vi "RFmxSpecAn Get Results Deployed(Harms).vi"(0 "SA Handle In":refnum<k21> caption="Instrument Handle In", 2 "# of Harms":i32=1 min=1 max=10, 5 "Center Freq (MHz) In":dbl, 11 "error in (no error)":errorcluster) -> (4 "SA Handle Out":refnum<k21> caption="Instrument Handle Out", 6 "Harms Results dBm":dbl[][](array[numeric]), 15 "error out":errorcluster)   [LabVIEW 2018]
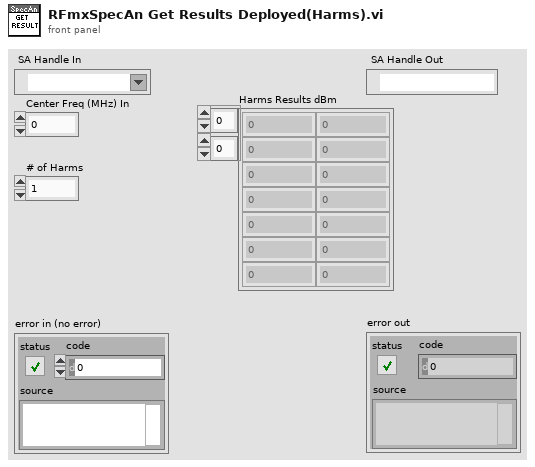
[diagram p1: front panel]
types:
  T1 = typedef "niRFmx Instrument Handle.ctl" = refnum<k21>
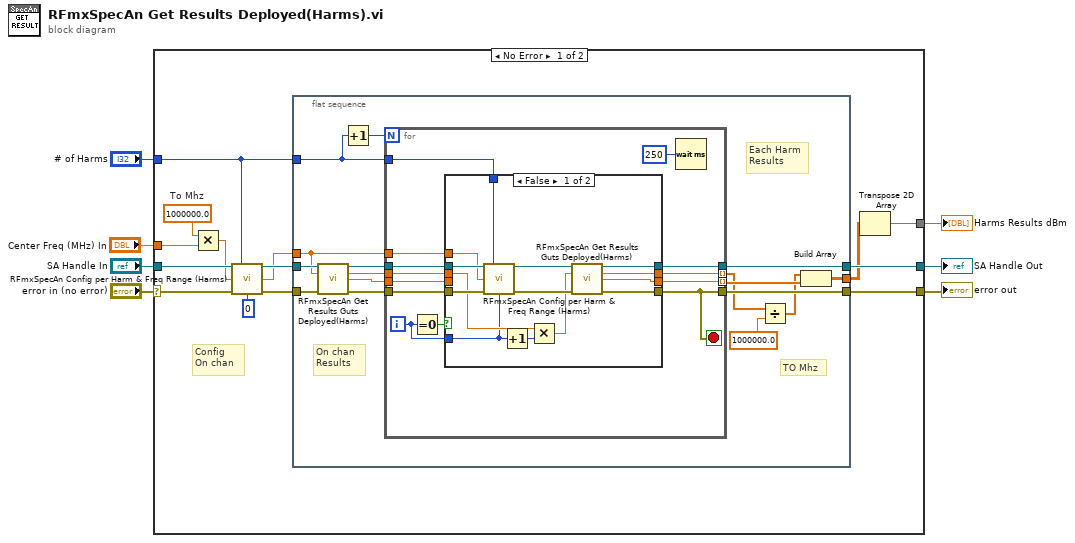
[diagram p0: block diagram]
diagram:
  n1 = case shown="No Error" "error in (no error)" {
    selector: "error in (no error)" -> [w14 w69]
    tunnel: "SA Handle In" -> [w21 w70]
    tunnel: [w13 w69] -> w5
    tunnel: [w20 w70] -> w4
    tunnel: "# of Harms" -> [w19 _]
    tunnel: "Center Freq (MHz) In" -> [w11 _]
    tunnel: [w8 _] -> w1
    frame No Error {
      w9 = 1000000.0  # To Mhz
      # "Config \nOn chan"
      n2 = Multiply(x=w9, y=w11) -> (x*y=w10:dbl)
      n3 = call "RFmxSpecAn Config per Harm & Freq Range (Harms).vi"("SA Handle In"=w21, "# of Harms"=w19, "Center Freq (Hz) In"=w10, "error in (no error)"=w14, "Meas Harm #"=u8 0) -> ("SA Handle Out"=w18:refnum<k21>, "Center Freq (Hz) Out"=w15:dbl, "error out"=w17:errorcluster)  [unwired: 8 in]
      n4 = flat-sequence {
        tunnel: w18 -> [w33]
        tunnel: w17 -> [w32]
        tunnel: [w37] -> w13
        tunnel: [w36] -> w20
        tunnel: w19 -> [w24]
        tunnel: [w28] -> w12
        tunnel: w15 -> [w23]
        frame #0 {
          # "TO Mhz"
          # "Each Harm\nResults"
          # "On chan \nResults"
          n5 = call "RFmxSpecAn Get Results Guts Deployed(Harms).vi"("Refnum in"=w33, "Center Freq (Hz)"=w23, "error in (no error)"=w32) -> ("Refnum out"=w30:T1, "Peak Frequency (Hz)"=w35:dbl, "Peak Amplitude"=w34:dbl, "error out"=w31:errorcluster)  [unwired: 9 in]
          n6 = Increment(x=w24) -> (x+1=w25:i32)
          n7 = for {
            N: w25 -> [_]
            tunnel: w30 -> [w50]
            tunnel: w31 -> [w49]
            tunnel: [w41] -> w37
            tunnel: [w48] -> w36
            tunnel: w35 -> [w46]
            tunnel: w34 -> [w45]
            tunnel: [w43] -> w29 mode=indexing
            tunnel: w24 -> [w42]
            tunnel: w23 -> [w39]
            tunnel: [w38] -> w22 mode=indexing
            i -> [w40]
            stop <- w41 stop-if-true
            n8 = Equal To 0?(x=w40) -> (x = 0?=w44:bool)
            n9 = case shown="False" w44 {
              tunnel: w50 -> [w59 w67]
              tunnel: w49 -> [w61 w68]
              tunnel: [w64 w68] -> w41
              tunnel: [w63 w67] -> w48
              tunnel: w46 -> [w54 w65]
              tunnel: w45 -> [_ w66]
              tunnel: [w62 w66] -> w43
              tunnel: w42 -> [w57 _]
              tunnel: w40 -> [w52 _]
              tunnel: w39 -> [w55 _]
              tunnel: [w51 w65] -> w38
              frame False {
                n10 = call "RFmxSpecAn Config per Harm & Freq Range (Harms).vi"("SA Handle In"=w59, "# of Harms"=w57, "Center Freq (Hz) In"=w55, "error in (no error)"=w61, "Meas Harm #"=w52) -> ("SA Handle Out"=w58:refnum<k21>, "error out"=w60:errorcluster)  [unwired: 8 in, 1 out]
                n11 = Increment(x=w52) -> (x+1=w53:i32)
                n12 = Multiply(x=w54, y=w53) -> (x*y=w56:dbl)
                n13 = call "RFmxSpecAn Get Results Guts Deployed(Harms).vi"("Refnum in"=w58, "Center Freq (Hz)"=w56, "error in (no error)"=w60) -> ("Refnum out"=w63:T1, "Peak Frequency (Hz)"=w51:dbl, "Peak Amplitude"=w62:dbl, "error out"=w64:errorcluster)  [unwired: 9 in]
              }
              frame True {
              }
            }
            n14 = Wait (ms)(milliseconds to wait=u32 250) -> ()  [unwired: 1 out]
          }
          n15 = Divide(x=w22, y=1000000.0) -> (x/y=w27:dbl[])
          n16 = Build Array(w27, w29) -> (w28:dbl[][])
        }
      }
      n17 = Transpose 2D Array(2D array=w12) -> (transposed array=w8:dbl[][])
    }
    frame Error {
    }
  }
  "error out" <- w5
  "SA Handle Out" <- w4
  "Harms Results dBm" <- w1
